vi "Build Project Tree.vi"(8 "error in (no error)":errorcluster, 9 "Include Dependencies?":bool, 10 "Project Index":u16, 11 "Message Maker in":refnum<class "Message Maker.lvclass">) -> (0 "error out":errorcluster, 2 "Messages out of Date?":bool, 3 "Message Maker out":refnum<class "Message Maker.lvclass">)   [LabVIEW 2023, in "Message Maker.lvclass"]
doc: "Populates the tree with the information about all actors in the project\n\nAuthor: Derek Trepanier\nCopyright: MGI 2015"
uses:
  Message Maker.lvclass
  Message Maker.lvclass/Message Maker.ctl
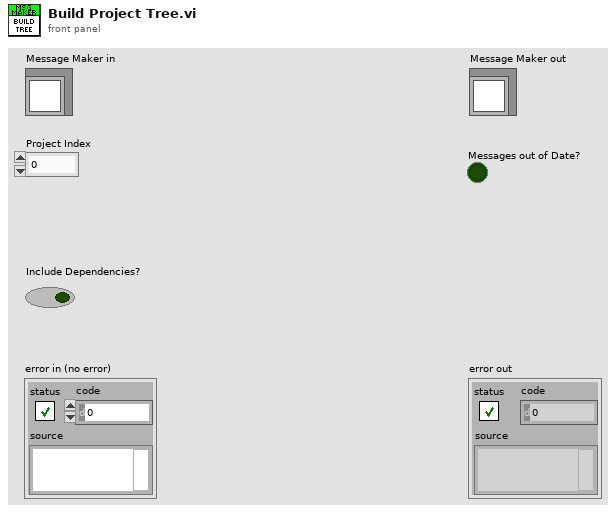
[diagram p1: front panel]
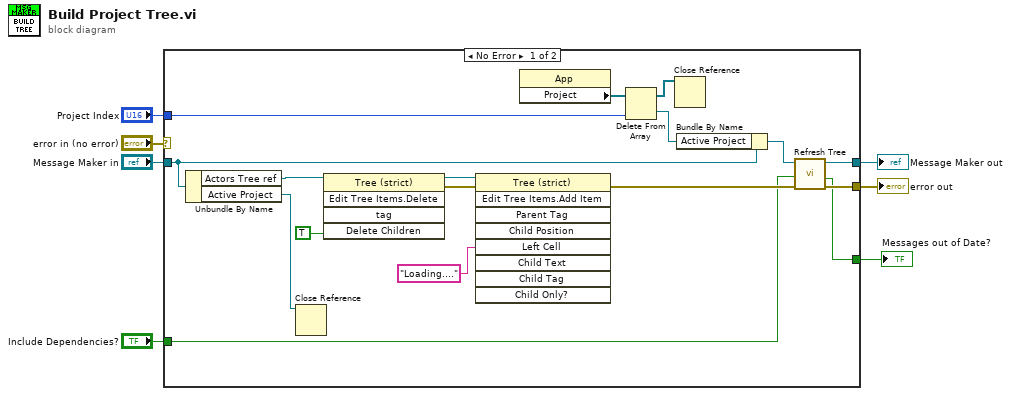
[diagram p0: block diagram]
diagram:
  n1 = case shown="No Error" "error in (no error)" {
    selector: "error in (no error)" -> [_ w26]
    tunnel: [w13 w26] -> w6
    tunnel: [w18 w25] -> w4
    tunnel: "Message Maker in" -> [w23 w25]
    tunnel: "Project Index" -> [w16 _]
    tunnel: "Include Dependencies?" -> [w9 _]
    tunnel: [w8 _] -> w1
    frame No Error {
      n2 = Unbundle By Name(w23) -> ("Actors Tree ref"=w20:refnum<vi>, "Active Project"=w12:refnum<vi>)
      n3 = Close Reference(reference=w12) -> ()  [unwired: 1 in, 1 out]
      n4 = invoke class="Tree (strict)" method="Edit Tree Items.Delete"(reference=w20, "Delete Children"=TRUE ("Delete Children?")) -> (reference out=w22:refnum<vi>, error out=w21:errorcluster)  [unwired: 3 in, 3 out]
      n5 = invoke class="Tree (strict)" method="Edit Tree Items.Add Item"(reference=w22, error in=w21, "Left Cell"="Loading...." ("Left Cell String")) -> (error out=w14:errorcluster)  [unwired: 6 in, 8 out]
      n6 = property class="App"() -> ("Project"=w17:refnum<vi>[])  [unwired: 2 in, 2 out]
      n7 = Delete From Array(array=w17, index=w16) -> (deleted portion=w10:refnum<vi>, array with subset deleted=w15:refnum<vi>[])  [unwired: 1 in]
      n8 = Close Reference(reference=w15) -> ()  [unwired: 1 in, 1 out]
      n9 = Bundle By Name(cluster=w23, "Active Project"=w10) -> (w11:refnum<class "Message Maker.lvclass">)
      n10 = call "Refresh Tree.vi"("error in (no error)"=w14, "Include Dependencies?"=w9, "Message Maker in"=w11) -> ("error out"=w13:errorcluster, "Messages out of date?"=w8:bool, "Message Maker out"=w18:refnum<class "Message Maker.lvclass">)  [unwired: 6 in]
    }
    frame Error {
    }
  }
  "error out" <- w6
  "Message Maker out" <- w4
  "Messages out of Date?" <- w1
